vi "ReadConfigurationFile_Algo.vi"(0 "Update":bool, 1 "Override Configuration file path":path=path "C:/Users/deeps/Desktop/Documentation/Final ZenGage V1.3.1/ZenGage V1.3.1 exe/Configuration file/Algorithm Parameters Override.json", 2 "Default Configuration file path":path=path "C:/Users/deeps/Desktop/Documentation/Final ZenGage V1.3.1/ZenGage V1.3.1 exe/Configuration file/Algorithm Parameters Default.json", 5 "DefaultVariant":variant, 7 "OutputClusterIn":T1={"Acknowledgement"={"Enqueuer"=refnum, "VIReference"=refnum, "VIName"=""}, "AllPartInfo"=[{"PartName"="", "NumberOfRacks"=0, "MeasurementIDsArray"=[], "MeasurementNamesArray"=[], "SpecValuesArray"=[]}], "PartInfo"={"PartName"="", "TotalCount"=0, "ReelCount"=0, "NumberOfRacks"=0, "MeasurementIDsArray"=[], "MeasurementNamesArray"=[], "SpecValuesArray"=[]}, "Result Cluster"={"Measurement Names Array"=[], "Pass-Fail Array"=[], "Measurement Values Array "=[], "Roi for overlay (Arrows) Array"=[], "Algo Type Array"=[], "Image Array"=[], "Clamp operations"=enum."Average Clamp", "  Search Direction "=[], "Images_Array_in"=[], "ResultPF"=FALSE, "Total Cluster Values"={"Total Fail"=0, "Total Pass"=0, "Total Count"=0}, "Reel Counter Cluster"={"Reel Fail"=0, "Reel Pass"=0, "Reel Count"=0}, "Tolerance  Array"=[], "Array of Cam Spec Control Bool"=[], "Control Pass Fail Array"=[], "Specification Pass Fail Array"=[], "Overlay Arrow Lines"=[], "Camera ID"=[], "Trigger count"=0, "Specification fail?"=FALSE}, "ErrorMessage"=""}, 9 "AlgoParameters":T6, 11 "error in":errorcluster) -> (4 "DefaultVariantOut":variant, 6 "OutputClusterOut":T1={"Acknowledgement"={"Enqueuer"=refnum, "VIReference"=refnum, "VIName"=""}, "AllPartInfo"=[], "PartInfo"={"PartName"="", "TotalCount"=0, "ReelCount"=0, "NumberOfRacks"=0, "MeasurementIDsArray"=[], "MeasurementNamesArray"=[], "SpecValuesArray"=[]}, "Result Cluster"={"Measurement Names Array"=[], "Pass-Fail Array"=[], "Measurement Values Array "=[], "Roi for overlay (Arrows) Array"=[], "Algo Type Array"=[], "Image Array"=[], "Clamp operations"=enum."Average Clamp", "  Search Direction "=[], "Images_Array_in"=[], "ResultPF"=FALSE, "Total Cluster Values"={"Total Fail"=0, "Total Pass"=0, "Total Count"=0}, "Reel Counter Cluster"={"Reel Fail"=0, "Reel Pass"=0, "Reel Count"=0}, "Tolerance  Array"=[], "Array of Cam Spec Control Bool"=[], "Control Pass Fail Array"=[], "Specification Pass Fail Array"=[], "Overlay Arrow Lines"=[], "Camera ID"=[], "Trigger count"=0, "Specification fail?"=FALSE}, "ErrorMessage"=""}, 8 "AllAlgoParameters":T6, 15 "error out":errorcluster)   [LabVIEW 2019, in "Algorithm.lvclass"]
uses:
  FrameworkOverrides/Algorithm.lvclass
  <vilib>/ActorFramework/Message Enqueuer/Message Enqueuer.lvclass
  Common/Controls/AllPartInfo.ctl
  Common/Controls/Acknowledgement.ctl
  Controls/OutputCluster.ctl
  Controls/Result Cluster.ctl
panel:
  out "JSON Variant 2":variant
  out "JSON Variant":variant
  out "Queried Cluster":variant
  out "Default JSON string":string
  out "Override JSON string":string
  out "Error Message":string
  out "Output Merged Cluster":variant
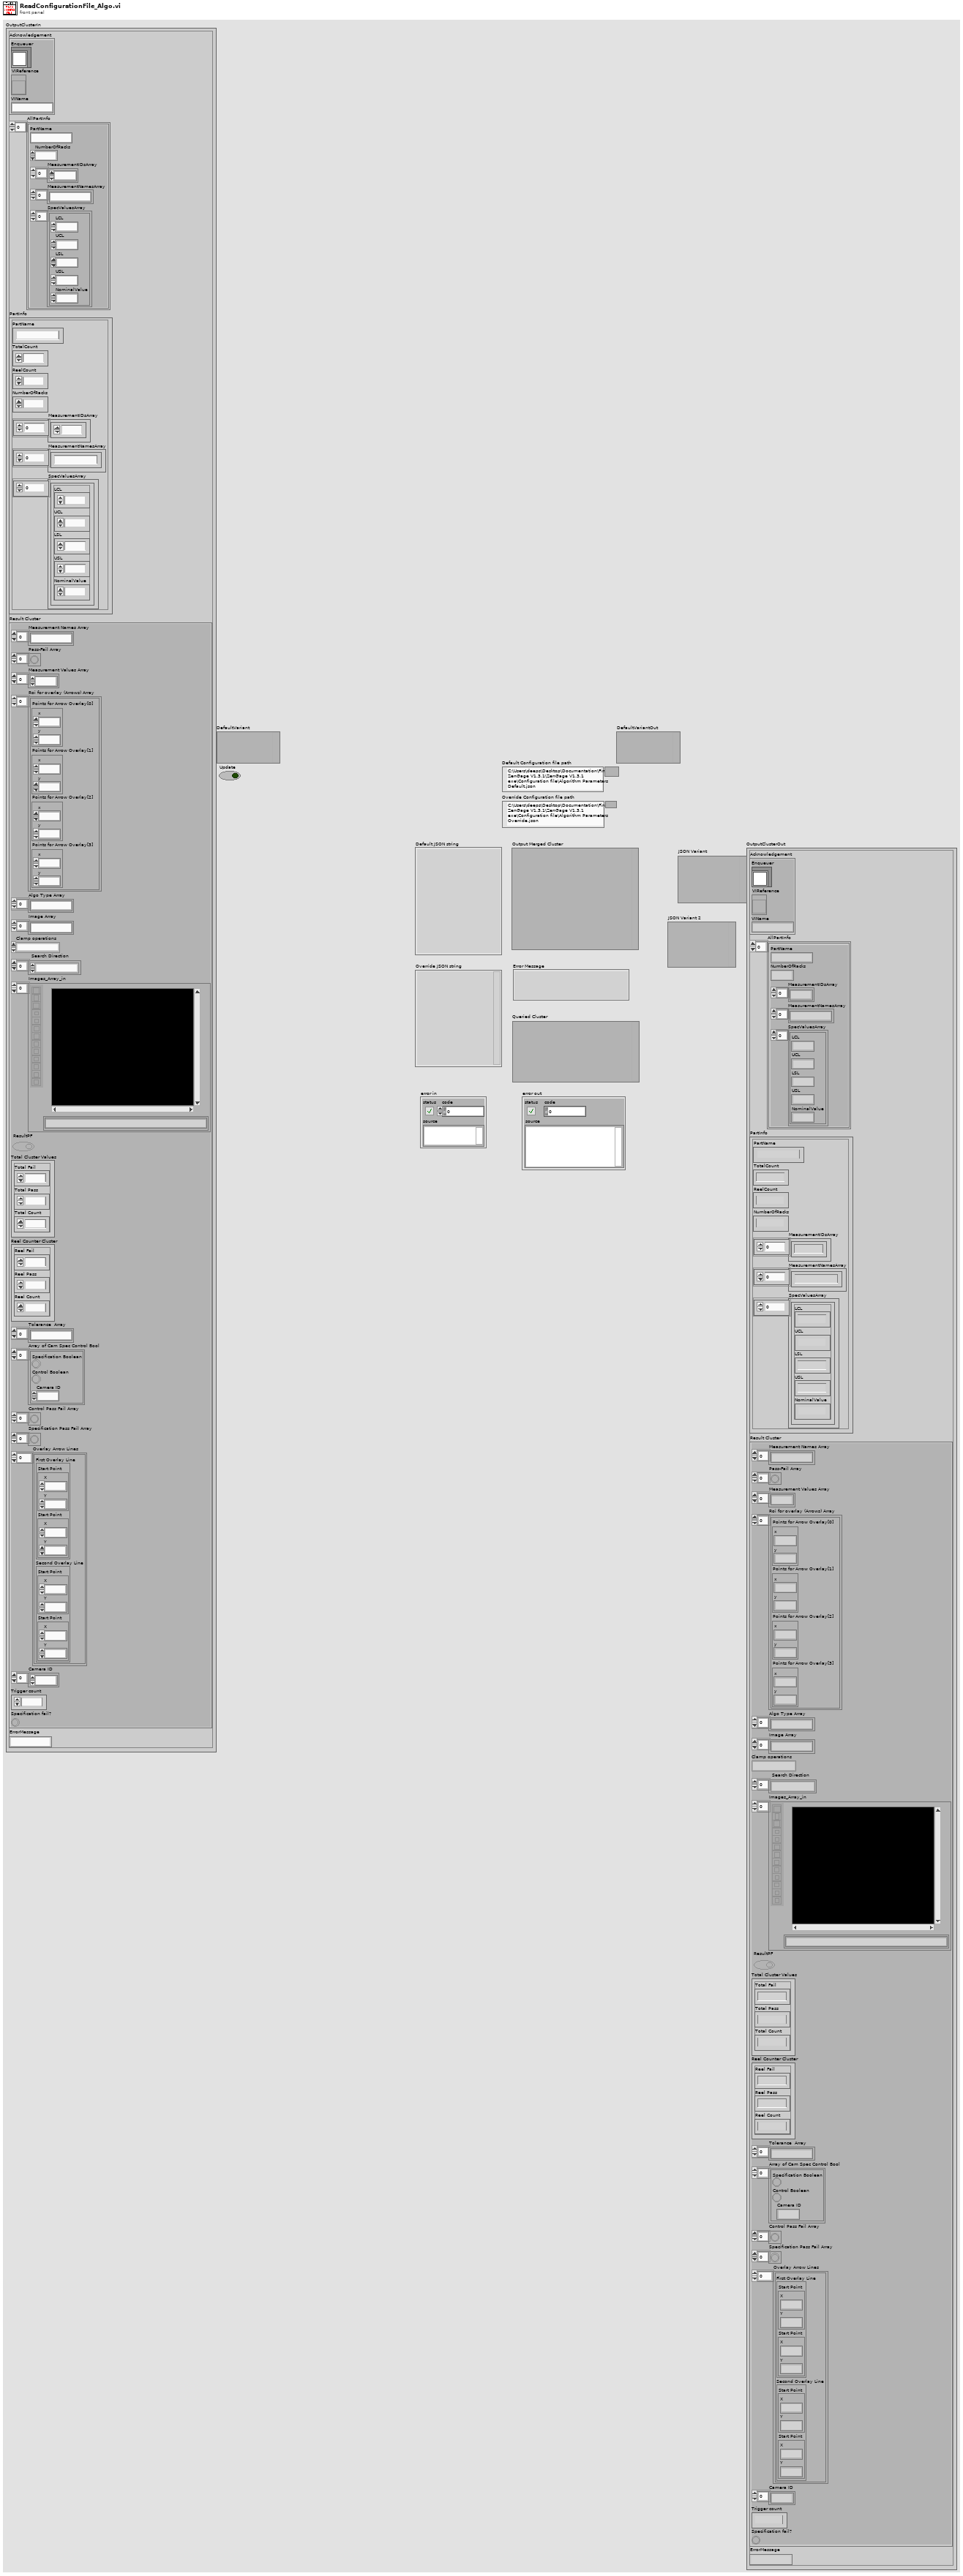
[diagram p1: front panel]
types:
  T1 = typedef "Algorithm.lvclass/OutputCluster.ctl" = cluster{"Acknowledgement":T2, "AllPartInfo":T3, "PartInfo":cluster{"PartName":string, "TotalCount":u64, "ReelCount":u64, "NumberOfRacks":u8, "MeasurementIDsArray":u16[], "MeasurementNamesArray":string[], "SpecValuesArray":cluster{"LCL":dbl, "UCL":dbl, "LSL":dbl, "USL":dbl, "NominalValue":dbl}[]}, "Result Cluster":T4, "ErrorMessage":string}
  T2 = typedef "Acknowledgement.ctl" = cluster{"Enqueuer":refnum<class "Message Enqueuer.lvclass">, "VIReference":refnum<vi>, "VIName":string}
  T3 = typedef "AllPartInfo.ctl" = cluster{"PartName":string, "NumberOfRacks":u8, "MeasurementIDsArray":u16[], "MeasurementNamesArray":string[], "SpecValuesArray":cluster{"LCL":dbl, "UCL":dbl, "LSL":dbl, "USL":dbl, "NominalValue":dbl}[]}[]
  T4 = typedef "Algorithm.lvclass/Result Cluster.ctl" = cluster{"Measurement Names Array":string[], "Pass-Fail Array":bool[], "Measurement Values Array ":dbl[], "Roi for overlay (Arrows) Array":cluster{"Points for Arrow Overlay[0]":cluster{"x":dbl, "y":dbl}, "Points for Arrow Overlay[1]":cluster{"x":dbl, "y":dbl}, "Points for Arrow Overlay[2]":cluster{"x":dbl, "y":dbl}, "Points for Arrow Overlay[3]":cluster{"x":dbl, "y":dbl}}[], "Algo Type Array":string[], "Image Array":string[], "Clamp operations":enum16{"Min Clamp", "Max Clamp", "Average Clamp"}, "  Search Direction ":enum16{"Left to Right", "Right to Left", "Top to Bottom", "Bottom to Top"}[], "Images_Array_in":T5[], "ResultPF":bool, "Total Cluster Values":cluster{"Total Fail":u64, "Total Pass":u64, "Total Count":u64}, "Reel Counter Cluster":cluster{"Reel Fail":u64, "Reel Pass":u64, "Reel Count":u64}, "Tolerance  Array":string[], "Array of Cam Spec Control Bool":cluster{"Specification Boolean":bool, "Control Boolean":bool, "Camera ID":i8}[], "Control Pass Fail Array":bool[], "Specification Pass Fail Array":bool[], "Overlay Arrow Lines":cluster{"First Overlay Line ":cluster{"Start Point":cluster{"X":sgl, "Y":sgl}, "Start Point":cluster{"X":sgl, "Y":sgl}}, "Second Overlay Line ":cluster{"Start Point":cluster{"X":sgl, "Y":sgl}, "Start Point":cluster{"X":sgl, "Y":sgl}}}[], "Camera ID":i8[], "Trigger count":i32, "Specification fail?":bool}
  T5 = typedef "IMAQ Image.ctl" = refnum<image>
  T6 = cluster{"PartsList":cluster{"Name":string, "ImageStreams":cluster{"ThreadName":string, "RackEnable":bool, "ThreadId":i32, "RackId":i32, "DifferenceParameter":i32, "SplitCameraIDs":i32[], "ImagingViews":cluster{"ViewName":string, "ViewEnable":bool, "ImageID":i32, "CameraID":i32, "CalibrationFilePath":string, "CalibImageFormat":string, "ReferenceCoordSystem":cluster{"Method":cluster{"Algo":string, "BaseReference":cluster{"OriginX":i32, "OriginY":i32, "Angle":dbl, "AxisReference":i32}}, "ROI1":cluster{"ROI":cluster{"Left":i32, "Top":i32, "Right":i32, "Bottom":i32, "Rotation":dbl}, "EdgeOptions":cluster{"EdgePolarity":i32, "KernelSize":i32, "Width":i32, "MinimumEdgeStrength":i32, "InterpolationType":i32, "DataProcessingMethod":i32}, "LineOptions":cluster{"NumberofLines":i32, "Type":i32, "MinScore":i32, "MaxScore":i32, "Orientation":i32, "AngleRange":i32, "AngleTolerance":i32, "StepSize":i32, "MinSNR":i32, "MinPoints":i32, "HoughIterations":i32}, "Process":i32, "StepSize":i32, "SearchDirection":i32, "CircleEdgeOptions":cluster{"SearchDirection":i32, "EdgeOptions":cluster{"EdgePolarity":i32, "KernelSize":i32, "Width":i32, "MinimumEdgeStrength":i32, "InterpolationType":i32, "DataProcessingMethod":i32}}, "CircleFitOptions":cluster{"Process":i32, "StepSize":i32, "MAxPixelRadius":i32}, "CircleSearchDirection":i32, "CurveParameters":cluster{"ExtractionMode":i32, "EdgeThreshold":i32, "EdgeFilterSize":i32, "MinLength":i32, "RowSearchStepSize":i32, "ColSearchStepSize":i32, "MaxEndpointGap":i32, "Closed":bool, "Subpixel":bool}, "MinimumMatchScore":i32, "CircleDescriptor":cluster{"MinRadius":i32, "MaxRadius":i32}, "EllipseDescriptor":cluster{"MinMajorRadius":i32, "MaxMajorRadius":i32, "MinMinorRadius":i32, "MaxMinorRadius":i32}, "ParallelLines":cluster{"First":i32, "Second":i32, "Third":i32}}[], "Name":string, "OverlayOptions":cluster{"OverlayEnable":bool, "OverlayText":string, "OverlayCoords":i32[], "OverlayAngle":i32, "OverlayTextSize":i32, "OverlayTextColor":string, "OverlayROI":bool, "OverlayRakeLine":bool, "OverlayPoints":bool}}, "CameraAngle":dbl[]}[]}[], "Measurements":cluster{"RackID":i32, "ImageID":i32, "CameraID":i32, "MeasurementId":i32, "Name":string, "AlgoName":string, "Type":string, "MeasurementEnable":bool, "AlgorithmSequence":cluster{"RefernceEdge":cluster{"Enable":bool, "Method":string, "RefROI":cluster{"Left":i32, "Top":i32, "Right":i32, "Bottom":i32, "Rotation":dbl}, "EdgeOptions":cluster{"EdgePoarity":i32, "KernelSize":i32, "Width":i32, "MinimumEdgeStrength":i32, "InterpolationType":i32, "DataProcessingMethod":i32}, "LineOptions":cluster{"NumberofLines":i32, "Type":i32, "MinScore":i32, "MaxScore":i32, "Orientation":i32, "AngleRange":i32, "AngleTolerance":i32, "StepSize":i32, "MinSNR":i32, "MinPoints":i32, "HoughIterations":i32}, "SearchDirection":i32}, "Measurement":cluster{"ROI1":cluster{"Enable":bool, "ROI":cluster{"Left":i32, "Top":i32, "Right":i32, "Bottom":i32, "Rotation":dbl}, "EdgeOptions":cluster{"EdgePoarity":i32, "KernelSize":i32, "Width":i32, "MinimumEdgeStrength":i32, "InterpolationType":i32, "DataProcessingMethod":i32}, "LineOptions":cluster{"NumberofLines":i32, "Type":i32, "MinScore":i32, "MaxScore":i32, "Orientation":i32, "AngleRange":i32, "AngleTolerance":i32, "StepSize":i32, "MinSNR":i32, "MinPoints":i32, "HoughIterations":i32}, "Process":i32, "StepSize":i32, "SearchDirection":i32, "CircleEdgeOptions":cluster{"SearchDirection":i32, "EdgeOptions":cluster{"EdgePoarity":i32, "KernelSize":i32, "Width":i32, "MinimumEdgeStrength":i32, "InterpolationType":i32, "DataProcessingMethod":i32}}, "CircleFitOptions":cluster{"Process":i32, "StepSize":i32, "MAxPixelRadius":dbl}, "CircleSearchDirection":i32, "CurveParameters":cluster{"ExtractionMode":i32, "EdgeThreshold":i32, "EdgeFilterSize":i32, "MinLength":i32, "RowSearchStepSize":i32, "ColSearchStepSize":i32, "MaxEndpointGap":i32, "Closed":bool, "Subpixel":bool}, "MinimumMatchScore":i32, "CircleDescriptor":cluster{"MinRadius":i32, "MaxRadius":i32}, "EllipseDescriptor":cluster{"MinMajorRadius":i32, "MaxMajorRadius":i32, "MinMinorRadius":i32, "MaxMinorRadius":i32}}, "ROI2":cluster{"Enable":bool, "ROI":cluster{"Left":i32, "Top":i32, "Right":i32, "Bottom":i32, "Rotation":dbl}, "EdgeOptions":cluster{"EdgePoarity":i32, "KernelSize":i32, "Width":i32, "MinimumEdgeStrength":i32, "InterpolationType":i32, "DataProcessingMethod":i32}, "LineOptions":cluster{"NumberofLines":i32, "Type":i32, "MinScore":i32, "MaxScore":i32, "Orientation":i32, "AngleRange":i32, "AngleTolerance":i32, "StepSize":i32, "MinSNR":i32, "MinPoints":i32, "HoughIterations":i32}, "Process":i32, "StepSize":i32, "SearchDirection":i32, "CircleEdgeOptions":cluster{"SearchDirection":i32, "EdgeOptions":cluster{"EdgePoarity":i32, "KernelSize":i32, "Width":i32, "MinimumEdgeStrength":i32, "InterpolationType":i32, "DataProcessingMethod":i32}}, "CircleFitOptions":cluster{"Process":i32, "StepSize":i32, "MAxPixelRadius":dbl}, "CircleSearchDirection":i32, "CurveParameters":cluster{"ExtractionMode":i32, "EdgeThreshold":i32, "EdgeFilterSize":i32, "MinLength":i32, "RowSearchStepSize":i32, "ColSearchStepSize":i32, "MaxEndpointGap":i32, "Closed":bool, "Subpixel":bool}, "MinimumMatchScore":i32, "CircleDescriptor":cluster{"MinRadius":i32, "MaxRadius":i32}, "EllipseDescriptor":cluster{"MinMajorRadius":i32, "MaxMajorRadius":i32, "MinMinorRadius":i32, "MaxMinorRadius":i32}}}}, "MathExpression":cluster{"Algorithm":string, "MathExpression":string, "ResultVariable":string}, "MathCorrectionParameters":cluster{"Radius":dbl, "CurlGap":dbl, "Thickness":dbl, "MeasurementIndices":i32[], "MathAlgoName":string, "MathAlgoFormula":string, "CorrectionForAngle":i32[], "NumericAray":i32[], "StringArray":string[]}, "ResultVariableCluster":cluster{"RVName":string, "RVSequence":string, "RVIndex":i32, "RVID":i32, "RVValue":dbl}, "CalibrationCoefficients":cluster{"A1":dbl, "A2":dbl, "A3":dbl}, "UserCalibCoefficients":cluster{"UserCorrectionLinearityCoeff":dbl, "UserCorrectionBiasCoeff":dbl}, "SpecValues":cluster{"LCL":dbl, "UCL":dbl, "LSL":dbl, "USL":dbl, "NominalValue":dbl}, "OverlayOptions":cluster{"OverlayEnable":bool, "OverlayText":string, "OverlayCoords":i32[], "OverlayAngle":i32, "OverlayTextSize":i32, "OverlayTextColor":string, "OverlayROI":bool, "OverlayRakeLine":bool, "OverlayPoints":bool}, "DatalogEnable":bool, "DisplayIcon":string}[]}[]}
  T7 = cluster{"Name":string, "ImageStreams":cluster{"ThreadName":string, "RackEnable":bool, "ThreadId":i32, "RackId":i32, "DifferenceParameter":i32, "SplitCameraIDs":i32[], "ImagingViews":cluster{"ViewName":string, "ViewEnable":bool, "ImageID":i32, "CameraID":i32, "CalibrationFilePath":string, "CalibImageFormat":string, "ReferenceCoordSystem":cluster{"Method":cluster{"Algo":string, "BaseReference":cluster{"OriginX":i32, "OriginY":i32, "Angle":dbl, "AxisReference":i32}}, "ROI1":cluster{"ROI":cluster{"Left":i32, "Top":i32, "Right":i32, "Bottom":i32, "Rotation":dbl}, "EdgeOptions":cluster{"EdgePolarity":i32, "KernelSize":i32, "Width":i32, "MinimumEdgeStrength":i32, "InterpolationType":i32, "DataProcessingMethod":i32}, "LineOptions":cluster{"NumberofLines":i32, "Type":i32, "MinScore":i32, "MaxScore":i32, "Orientation":i32, "AngleRange":i32, "AngleTolerance":i32, "StepSize":i32, "MinSNR":i32, "MinPoints":i32, "HoughIterations":i32}, "Process":i32, "StepSize":i32, "SearchDirection":i32, "CircleEdgeOptions":cluster{"SearchDirection":i32, "EdgeOptions":cluster{"EdgePolarity":i32, "KernelSize":i32, "Width":i32, "MinimumEdgeStrength":i32, "InterpolationType":i32, "DataProcessingMethod":i32}}, "CircleFitOptions":cluster{"Process":i32, "StepSize":i32, "MAxPixelRadius":i32}, "CircleSearchDirection":i32, "CurveParameters":cluster{"ExtractionMode":i32, "EdgeThreshold":i32, "EdgeFilterSize":i32, "MinLength":i32, "RowSearchStepSize":i32, "ColSearchStepSize":i32, "MaxEndpointGap":i32, "Closed":bool, "Subpixel":bool}, "MinimumMatchScore":i32, "CircleDescriptor":cluster{"MinRadius":i32, "MaxRadius":i32}, "EllipseDescriptor":cluster{"MinMajorRadius":i32, "MaxMajorRadius":i32, "MinMinorRadius":i32, "MaxMinorRadius":i32}, "ParallelLines":cluster{"First":i32, "Second":i32, "Third":i32}}[], "Name":string, "OverlayOptions":cluster{"OverlayEnable":bool, "OverlayText":string, "OverlayCoords":i32[], "OverlayAngle":i32, "OverlayTextSize":i32, "OverlayTextColor":string, "OverlayROI":bool, "OverlayRakeLine":bool, "OverlayPoints":bool}}, "CameraAngle":dbl[]}[]}[], "Measurements":cluster{"RackID":i32, "ImageID":i32, "CameraID":i32, "MeasurementId":i32, "Name":string, "AlgoName":string, "Type":string, "MeasurementEnable":bool, "AlgorithmSequence":cluster{"RefernceEdge":cluster{"Enable":bool, "Method":string, "RefROI":cluster{"Left":i32, "Top":i32, "Right":i32, "Bottom":i32, "Rotation":dbl}, "EdgeOptions":cluster{"EdgePoarity":i32, "KernelSize":i32, "Width":i32, "MinimumEdgeStrength":i32, "InterpolationType":i32, "DataProcessingMethod":i32}, "LineOptions":cluster{"NumberofLines":i32, "Type":i32, "MinScore":i32, "MaxScore":i32, "Orientation":i32, "AngleRange":i32, "AngleTolerance":i32, "StepSize":i32, "MinSNR":i32, "MinPoints":i32, "HoughIterations":i32}, "SearchDirection":i32}, "Measurement":cluster{"ROI1":cluster{"Enable":bool, "ROI":cluster{"Left":i32, "Top":i32, "Right":i32, "Bottom":i32, "Rotation":dbl}, "EdgeOptions":cluster{"EdgePoarity":i32, "KernelSize":i32, "Width":i32, "MinimumEdgeStrength":i32, "InterpolationType":i32, "DataProcessingMethod":i32}, "LineOptions":cluster{"NumberofLines":i32, "Type":i32, "MinScore":i32, "MaxScore":i32, "Orientation":i32, "AngleRange":i32, "AngleTolerance":i32, "StepSize":i32, "MinSNR":i32, "MinPoints":i32, "HoughIterations":i32}, "Process":i32, "StepSize":i32, "SearchDirection":i32, "CircleEdgeOptions":cluster{"SearchDirection":i32, "EdgeOptions":cluster{"EdgePoarity":i32, "KernelSize":i32, "Width":i32, "MinimumEdgeStrength":i32, "InterpolationType":i32, "DataProcessingMethod":i32}}, "CircleFitOptions":cluster{"Process":i32, "StepSize":i32, "MAxPixelRadius":dbl}, "CircleSearchDirection":i32, "CurveParameters":cluster{"ExtractionMode":i32, "EdgeThreshold":i32, "EdgeFilterSize":i32, "MinLength":i32, "RowSearchStepSize":i32, "ColSearchStepSize":i32, "MaxEndpointGap":i32, "Closed":bool, "Subpixel":bool}, "MinimumMatchScore":i32, "CircleDescriptor":cluster{"MinRadius":i32, "MaxRadius":i32}, "EllipseDescriptor":cluster{"MinMajorRadius":i32, "MaxMajorRadius":i32, "MinMinorRadius":i32, "MaxMinorRadius":i32}}, "ROI2":cluster{"Enable":bool, "ROI":cluster{"Left":i32, "Top":i32, "Right":i32, "Bottom":i32, "Rotation":dbl}, "EdgeOptions":cluster{"EdgePoarity":i32, "KernelSize":i32, "Width":i32, "MinimumEdgeStrength":i32, "InterpolationType":i32, "DataProcessingMethod":i32}, "LineOptions":cluster{"NumberofLines":i32, "Type":i32, "MinScore":i32, "MaxScore":i32, "Orientation":i32, "AngleRange":i32, "AngleTolerance":i32, "StepSize":i32, "MinSNR":i32, "MinPoints":i32, "HoughIterations":i32}, "Process":i32, "StepSize":i32, "SearchDirection":i32, "CircleEdgeOptions":cluster{"SearchDirection":i32, "EdgeOptions":cluster{"EdgePoarity":i32, "KernelSize":i32, "Width":i32, "MinimumEdgeStrength":i32, "InterpolationType":i32, "DataProcessingMethod":i32}}, "CircleFitOptions":cluster{"Process":i32, "StepSize":i32, "MAxPixelRadius":dbl}, "CircleSearchDirection":i32, "CurveParameters":cluster{"ExtractionMode":i32, "EdgeThreshold":i32, "EdgeFilterSize":i32, "MinLength":i32, "RowSearchStepSize":i32, "ColSearchStepSize":i32, "MaxEndpointGap":i32, "Closed":bool, "Subpixel":bool}, "MinimumMatchScore":i32, "CircleDescriptor":cluster{"MinRadius":i32, "MaxRadius":i32}, "EllipseDescriptor":cluster{"MinMajorRadius":i32, "MaxMajorRadius":i32, "MinMinorRadius":i32, "MaxMinorRadius":i32}}}}, "MathExpression":cluster{"Algorithm":string, "MathExpression":string, "ResultVariable":string}, "MathCorrectionParameters":cluster{"Radius":dbl, "CurlGap":dbl, "Thickness":dbl, "MeasurementIndices":i32[], "MathAlgoName":string, "MathAlgoFormula":string, "CorrectionForAngle":i32[], "NumericAray":i32[], "StringArray":string[]}, "ResultVariableCluster":cluster{"RVName":string, "RVSequence":string, "RVIndex":i32, "RVID":i32, "RVValue":dbl}, "CalibrationCoefficients":cluster{"A1":dbl, "A2":dbl, "A3":dbl}, "UserCalibCoefficients":cluster{"UserCorrectionLinearityCoeff":dbl, "UserCorrectionBiasCoeff":dbl}, "SpecValues":cluster{"LCL":dbl, "UCL":dbl, "LSL":dbl, "USL":dbl, "NominalValue":dbl}, "OverlayOptions":cluster{"OverlayEnable":bool, "OverlayText":string, "OverlayCoords":i32[], "OverlayAngle":i32, "OverlayTextSize":i32, "OverlayTextColor":string, "OverlayROI":bool, "OverlayRakeLine":bool, "OverlayPoints":bool}, "DatalogEnable":bool, "DisplayIcon":string}[]}[]
  T8 = cluster{"PartName":string, "NumberOfRacks":u8, "MeasurementIDsArray":u16[], "MeasurementNamesArray":string[], "SpecValuesArray":cluster{"LCL":dbl, "UCL":dbl, "LSL":dbl, "USL":dbl, "NominalValue":dbl}[]}
  T9 = cluster{"PartName":string, "NumberOfRacks":u8, "MeasurementIDsArray":u16[], "MeasurementNamesArray":string[], "SpecValuesArray":cluster{"LCL":dbl, "UCL":dbl, "LSL":dbl, "USL":dbl, "NominalValue":dbl}[]}[]
  T10 = cluster{"RackID":i32, "ImageID":i32, "CameraID":i32, "MeasurementId":i32, "Name":string, "AlgoName":string, "Type":string, "MeasurementEnable":bool, "AlgorithmSequence":cluster{"RefernceEdge":cluster{"Enable":bool, "Method":string, "RefROI":cluster{"Left":i32, "Top":i32, "Right":i32, "Bottom":i32, "Rotation":dbl}, "EdgeOptions":cluster{"EdgePoarity":i32, "KernelSize":i32, "Width":i32, "MinimumEdgeStrength":i32, "InterpolationType":i32, "DataProcessingMethod":i32}, "LineOptions":cluster{"NumberofLines":i32, "Type":i32, "MinScore":i32, "MaxScore":i32, "Orientation":i32, "AngleRange":i32, "AngleTolerance":i32, "StepSize":i32, "MinSNR":i32, "MinPoints":i32, "HoughIterations":i32}, "SearchDirection":i32}, "Measurement":cluster{"ROI1":cluster{"Enable":bool, "ROI":cluster{"Left":i32, "Top":i32, "Right":i32, "Bottom":i32, "Rotation":dbl}, "EdgeOptions":cluster{"EdgePoarity":i32, "KernelSize":i32, "Width":i32, "MinimumEdgeStrength":i32, "InterpolationType":i32, "DataProcessingMethod":i32}, "LineOptions":cluster{"NumberofLines":i32, "Type":i32, "MinScore":i32, "MaxScore":i32, "Orientation":i32, "AngleRange":i32, "AngleTolerance":i32, "StepSize":i32, "MinSNR":i32, "MinPoints":i32, "HoughIterations":i32}, "Process":i32, "StepSize":i32, "SearchDirection":i32, "CircleEdgeOptions":cluster{"SearchDirection":i32, "EdgeOptions":cluster{"EdgePoarity":i32, "KernelSize":i32, "Width":i32, "MinimumEdgeStrength":i32, "InterpolationType":i32, "DataProcessingMethod":i32}}, "CircleFitOptions":cluster{"Process":i32, "StepSize":i32, "MAxPixelRadius":dbl}, "CircleSearchDirection":i32, "CurveParameters":cluster{"ExtractionMode":i32, "EdgeThreshold":i32, "EdgeFilterSize":i32, "MinLength":i32, "RowSearchStepSize":i32, "ColSearchStepSize":i32, "MaxEndpointGap":i32, "Closed":bool, "Subpixel":bool}, "MinimumMatchScore":i32, "CircleDescriptor":cluster{"MinRadius":i32, "MaxRadius":i32}, "EllipseDescriptor":cluster{"MinMajorRadius":i32, "MaxMajorRadius":i32, "MinMinorRadius":i32, "MaxMinorRadius":i32}}, "ROI2":cluster{"Enable":bool, "ROI":cluster{"Left":i32, "Top":i32, "Right":i32, "Bottom":i32, "Rotation":dbl}, "EdgeOptions":cluster{"EdgePoarity":i32, "KernelSize":i32, "Width":i32, "MinimumEdgeStrength":i32, "InterpolationType":i32, "DataProcessingMethod":i32}, "LineOptions":cluster{"NumberofLines":i32, "Type":i32, "MinScore":i32, "MaxScore":i32, "Orientation":i32, "AngleRange":i32, "AngleTolerance":i32, "StepSize":i32, "MinSNR":i32, "MinPoints":i32, "HoughIterations":i32}, "Process":i32, "StepSize":i32, "SearchDirection":i32, "CircleEdgeOptions":cluster{"SearchDirection":i32, "EdgeOptions":cluster{"EdgePoarity":i32, "KernelSize":i32, "Width":i32, "MinimumEdgeStrength":i32, "InterpolationType":i32, "DataProcessingMethod":i32}}, "CircleFitOptions":cluster{"Process":i32, "StepSize":i32, "MAxPixelRadius":dbl}, "CircleSearchDirection":i32, "CurveParameters":cluster{"ExtractionMode":i32, "EdgeThreshold":i32, "EdgeFilterSize":i32, "MinLength":i32, "RowSearchStepSize":i32, "ColSearchStepSize":i32, "MaxEndpointGap":i32, "Closed":bool, "Subpixel":bool}, "MinimumMatchScore":i32, "CircleDescriptor":cluster{"MinRadius":i32, "MaxRadius":i32}, "EllipseDescriptor":cluster{"MinMajorRadius":i32, "MaxMajorRadius":i32, "MinMinorRadius":i32, "MaxMinorRadius":i32}}}}, "MathExpression":cluster{"Algorithm":string, "MathExpression":string, "ResultVariable":string}, "MathCorrectionParameters":cluster{"Radius":dbl, "CurlGap":dbl, "Thickness":dbl, "MeasurementIndices":i32[], "MathAlgoName":string, "MathAlgoFormula":string, "CorrectionForAngle":i32[], "NumericAray":i32[], "StringArray":string[]}, "ResultVariableCluster":cluster{"RVName":string, "RVSequence":string, "RVIndex":i32, "RVID":i32, "RVValue":dbl}, "CalibrationCoefficients":cluster{"A1":dbl, "A2":dbl, "A3":dbl}, "UserCalibCoefficients":cluster{"UserCorrectionLinearityCoeff":dbl, "UserCorrectionBiasCoeff":dbl}, "SpecValues":cluster{"LCL":dbl, "UCL":dbl, "LSL":dbl, "USL":dbl, "NominalValue":dbl}, "OverlayOptions":cluster{"OverlayEnable":bool, "OverlayText":string, "OverlayCoords":i32[], "OverlayAngle":i32, "OverlayTextSize":i32, "OverlayTextColor":string, "OverlayROI":bool, "OverlayRakeLine":bool, "OverlayPoints":bool}, "DatalogEnable":bool, "DisplayIcon":string}[]
  T11 = cluster{"LCL":dbl, "UCL":dbl, "LSL":dbl, "USL":dbl, "NominalValue":dbl}
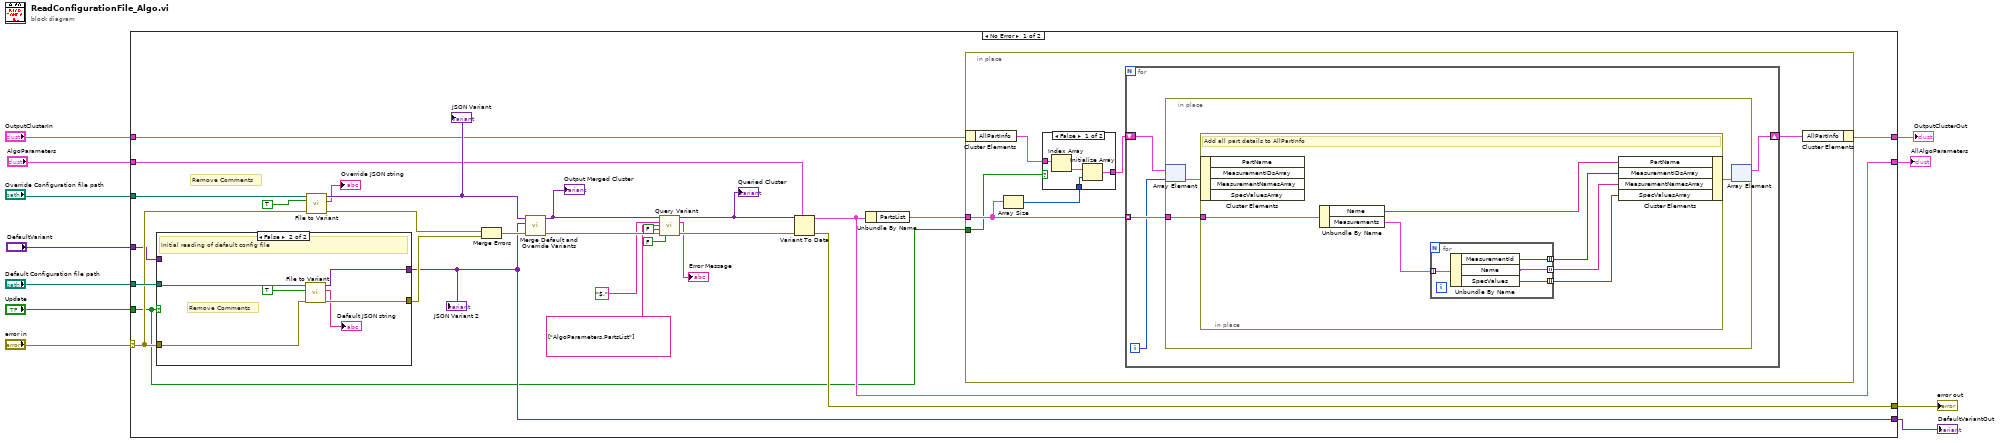
[diagram p0: block diagram]
diagram:
  n1 = case shown="No Error" "error in" {
    selector: "error in" -> [w24 w77]
    tunnel: "Override Configuration file path" -> [w37 _]
    tunnel: "Default Configuration file path" -> [w36 _]
    tunnel: [w31 w77] -> w9
    tunnel: "OutputClusterIn" -> [w23 w78]
    tunnel: [w22 w78] -> w4
    tunnel: "AlgoParameters" -> [w18 w76]
    tunnel: [w21 w76] -> w5
    tunnel: "Update" -> [w12 _]
    tunnel: "DefaultVariant" -> [w16 w75]
    tunnel: [w15 w75] -> w1
    frame No Error {
      # "Remove Comments"
      n2 = case shown="False" w12 {
        tunnel: w36 -> [_ w45]
        tunnel: [w39 w44] -> w15
        tunnel: [w40 w43] -> w33
        tunnel: w24 -> [w40 w42]
        tunnel: w16 -> [w39 _]
        frame True {
          # "Update case"
        }
        frame False {
          # "Remove Comments"
          # "Initial reading of default config file"
          n3 = call <vilib>:"File to Variant.vi"("JSON FilePath"=w45, "Remove Comments?"=TRUE, "error in (no error)"=w42) -> ("JSON Variant"=w44:variant, "Error message out"=→"Default JSON string":string, "error out"=w43:errorcluster)  [unwired: 5 in]
        }
      }
      "JSON Variant 2" <- w15
      n4 = call <vilib>:"File to Variant.vi"("JSON FilePath"=w37, "Remove Comments?"=TRUE, "error in (no error)"=w24) -> ("JSON Variant"=w35:variant, "Error message out"=→"Override JSON string":string, "error out"=w32:errorcluster)  [unwired: 5 in]
      "JSON Variant" <- w35
      n5 = Merge Errors(w32, w33) -> (w34:errorcluster)
      n6 = call <vilib>:"Merge Default and Override Variants.vi"("error in (no error)"=w34, "Default VCluster"=w15, "Override VCluster"=w35) -> ("error out"=w30:errorcluster, "Output Merged Cluster"=w20:variant)  [unwired: 7 in]
      "Output Merged Cluster" <- w20
      n7 = call <vilib>:"Query Variant.vi"("VCluster in"=w20, "basePath in"="$.", "pathList"=string[] ["AlgoParameters.PartsList"], "Reorder\nqueried\nvariants?"=FALSE ("Reorder\nqueried\nvariants?"), "error IO"=w30, "Include\n2D array?"=FALSE ("Include\n2D array?")) -> ("VCluster\n out"=w19:variant, "Error Message"=→"Error Message":string, "error out"=w29:errorcluster)  [unwired: 6 in, 1 out]
      "Queried Cluster" <- w19
      n8 = Variant To Data(error in=w29, type=w18, Variant=w19) -> (data=w21:T6, error out=w31:errorcluster)
      n9 = Unbundle By Name(w21) -> ("PartsList"=w25:T7)
      n10 = in-place {
        in-place-border: w25 -> [w50]
        in-place-border: w12 -> [w48]
        n11 = in-place-cluster #1(w23) -> ("AllPartInfo"=w51:T3)
        n12 = Array Size(array=w50) -> (size(s)=w49:i32)
        n13 = case shown="False" w48 {
          tunnel: w51 -> [w55 w57]
          tunnel: w49 -> [w54 _]
          tunnel: [w53 w57] -> w47
          frame False {
            n14 = Index Array(array=w55) -> (element=w56:T8)  [unwired: 1 in]
            n15 = Initialize Array(w56, w54) -> (w53:T9)
          }
          frame True {
          }
        }
        n16 = for {
          tunnel: w50 -> [w61] mode=indexing
          shift-right: [w58] -> w52
          shift-left: w47 -> [w60]
          i -> [w59]
          n17 = in-place {
            in-place-border: w61 -> [w64]
            n18 = in-place-array #2(w60, w59) -> (w63:T8)
            n19 = in-place {
              in-place-border: w64 -> [w70]
              # "Add all part details to AllPartInfo"
              n20 = in-place-cluster #3(w63) -> ()  [unwired: 4 out]
              n21 = Unbundle By Name(w70) -> ("Name"=w66:string, "Measurements"=w69:T10)
              n22 = for {
                tunnel: w69 -> [w74] mode=indexing
                tunnel: [w73] -> w67 mode=indexing
                tunnel: [w72] -> w68 mode=indexing
                tunnel: [w71] -> w65 mode=indexing
                n23 = Unbundle By Name(w74) -> ("MeasurementId"=w73:i32, "Name"=w72:string, "SpecValues"=w71:T11)
              }
              n24 = in-place-cluster #3("PartName"=w66, "MeasurementIDsArray"=w67, "MeasurementNamesArray"=w68, "SpecValuesArray"=w65) -> (w62:T8)
            }
            n25 = in-place-array #2(w62) -> (w58:T3)  [unwired: 1 out]
          }
        }
        n26 = in-place-cluster #1("AllPartInfo"=w52) -> (w22:T1)
      }
    }
    frame Error {
    }
  }
  "OutputClusterOut" <- w4
  "AllAlgoParameters" <- w5
  "error out" <- w9
  "DefaultVariantOut" <- w1
